vi "GetHGFunctionLookupTable.vi"(11 "G":dbl) -> (2 "Integrated Distribution":cluster{dbl[], dbl[]}(graph), 3 "Normalized Distribution":cluster{dbl[], dbl[]}(graph))   [LabVIEW 2019]
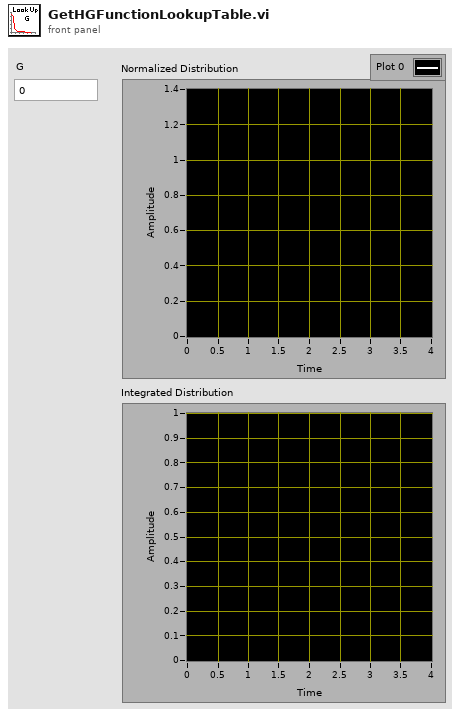
[diagram p1: front panel]
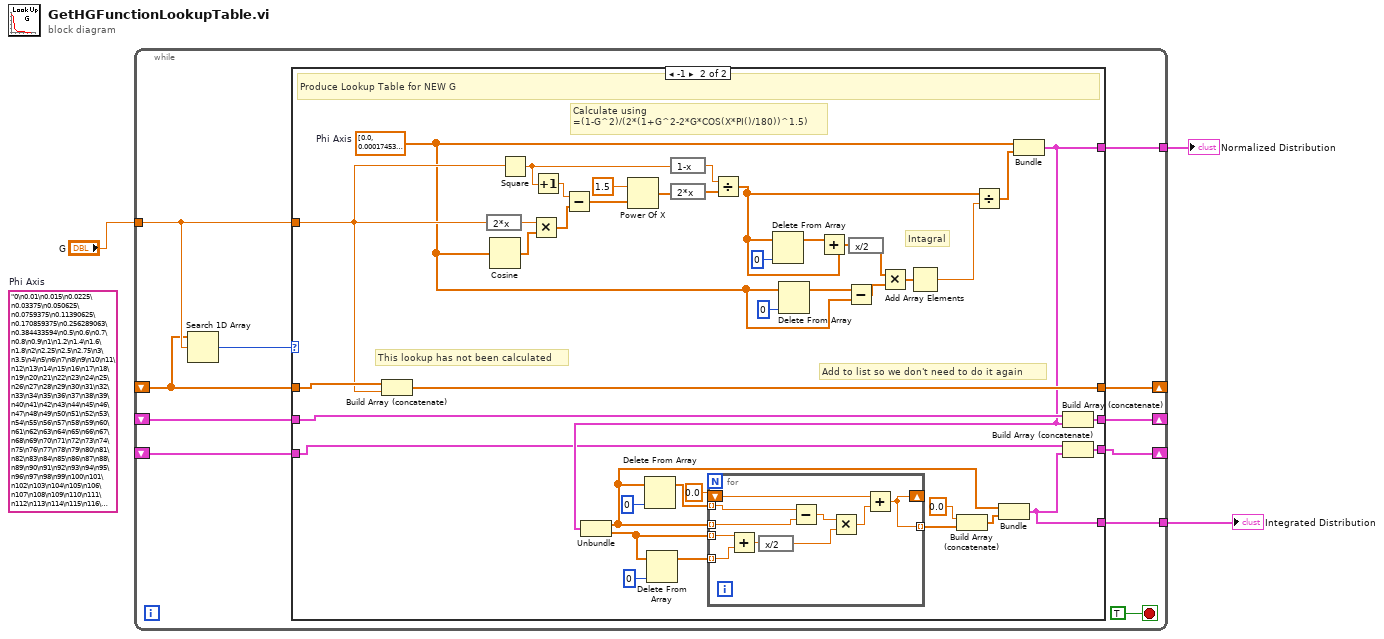
[diagram p0: block diagram]
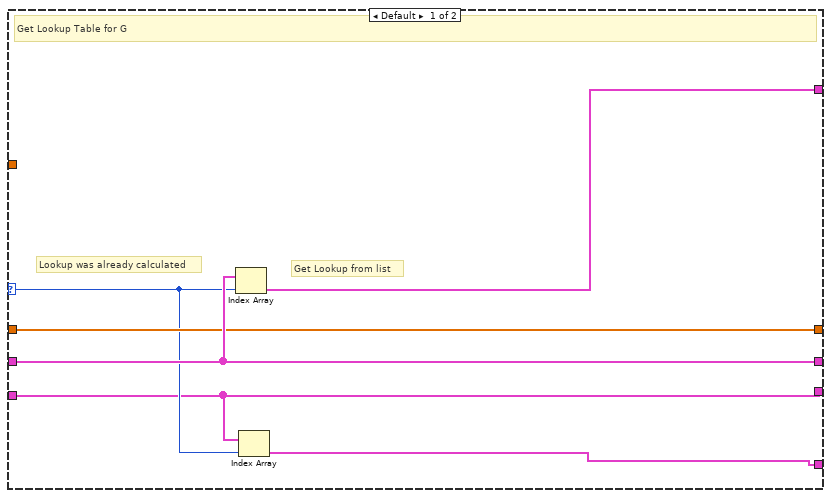
[diagram p2: hidden frame]
diagram:
  (unwired) "0\n0.01\n0.015\n0.0225\n0.03375\n0.050625\n0.0759375\n0.11390625\n0.170859375\n0.256289063\n0.384433594\n0.5\n0.6\n0.7\n0.8\n0.9\n1\n1.2\n1.4\n1.6\n1.8\n2\n2.25\n2.5\n2.75\n3\n3.5\n4\n5\n6\n7\n8\n9\n10\n11\n12\n13\n14\n15\n16\n17\n18\n19\n20\n21\n22\n23\n24\n25\n26\n27\n28\n29\n30\n31\n32\n33\n34\n35\n36\n37\n38\n39\n40\n41\n42\n43\n44\n45\n46\n47\n48\n49\n50\n51\n52\n53\n54\n55\n56\n57\n58\n59\n60\n61\n62\n63\n64\n65\n66\n67\n68\n69\n70\n71\n72\n73\n74\n75\n76\n77\n78\n79\n80\n81\n82\n83\n84\n85\n86\n87\n88\n89\n90\n91\n92\n93\n94\n95\n96\n97\n98\n99\n100\n101\n102\n103\n104\n105\n106\n107\n108\n109\n110\n111\n112\n113\n114\n115\n116\n117\n118\n119\n120\n121\n122\n123\n124\n125\n126\n127\n128\n129\n130\n131\n132\n133\n134\n135\n136\n137\n138\n139\n140\n141\n142\n143\n144\n145\n146\n147\n148\n149\n150\n151\n152\n153\n154\n155\n156\n157\n158\n159\n160\n161\n162\n163\n164\n165\n166\n167\n168\n169\n170\n171\n172\n173\n174\n175\n176\n177\n178\n179\n180\n"  # Phi Axis
  n1 = while {
    tunnel: [w14] -> w3
    shift-right: [w6] -> _
    shift-left: _ -> [w11]
    tunnel: "G" -> [w13]
    shift-right: [w5] -> _
    shift-left: _ -> [w10]
    tunnel: [w8] -> w1
    shift-right: [w4] -> _
    shift-left: _ -> [w7]
    stop <- TRUE stop-if-true
    n2 = Search 1D Array(1D array=w11, element=w13) -> (index of element=w12:i32)  [unwired: 1 in]
    n3 = case shown="-1" w12 {
      selector: w12 -> [w17 _]
      tunnel: [w20 w34] -> w14
      tunnel: w13 -> [_ w48]
      tunnel: w11 -> [w18 w50]
      tunnel: [w18 w49] -> w6
      tunnel: [w19 w47] -> w5
      tunnel: w10 -> [w19 w46]
      tunnel: [w15 w23] -> w8
      tunnel: [w16 w22] -> w4
      tunnel: w7 -> [w16 w21]
      frame Default {
        # "Get Lookup from list"
        # "Lookup was already calculated"
        # "Get Lookup Table for G"
        n4 = Index Array(array=w19, index=w17) -> (element=w20:cluster{"Phi Axis":dbl[], dbl[]})
        n5 = Index Array(array=w16, index=w17) -> (element=w15:cluster{"Phi Axis":dbl[], dbl[]})
      }
      frame -1 {
        w36 = dbl[] [0.0, 0.00017453292519943296, 0.0002617993877991494, 0.00039269908169872416, 0.0005890486225480862, 0.0008835729338221294, 0.001325359400733194, 0.001988039101099791, 0.0029820586516496866, 0.004473087986201175, 0.006709631970575117, 0.008726646259971648, 0.010471975511965976, 0.012217304763960306, 0.013962634015954637, 0.015707963267948967, 0.017453292519943295, 0.020943951023931952, 0.024434609527920613, 0.027925268031909273, 0.031415926535897934, 0.03490658503988659, 0.039269908169872414, 0.04363323129985824, 0.04799655442984406, 0.05235987755982988, 0.061086523819801536, 0.06981317007977318, 0.08726646259971647, 0.10471975511965977, 0.12217304763960307, 0.13962634015954636, 0.15707963267948966, 0.17453292519943295, 0.19198621771937624, 0.20943951023931953, 0.22689280275926285, 0.24434609527920614, 0.2617993877991494, 0.2792526803190927, 0.29670597283903605, 0.3141592653589793, 0.3316125578789226, 0.3490658503988659, 0.3665191429188092, 0.3839724354387525, 0.40142572795869574, 0.41887902047863906, 0.4363323129985824, 0.4537856055185257, 0.47123889803846897, 0.4886921905584123, 0.5061454830783556, 0.5235987755982988, 0.5410520681182421, 0.5585053606381855, 0.5759586531581288, 0.5934119456780721, 0.6108652381980153, 0.6283185307179586, 0.6457718232379019, 0.6632251157578452, 0.6806784082777885, 0.6981317007977318, 0.715584993317675, 0.7330382858376184, 0.7504915783575616, 0.767944870877505, 0.7853981633974483, 0.8028514559173915, 0.8203047484373349, 0.8377580409572781, 0.8552113334772214, 0.8726646259971648, 0.890117918517108, 0.9075712110370514, 0.9250245035569946, 0.9424777960769379, 0.9599310885968813, 0.9773843811168246, 0.9948376736367678, 1.0122909661567112, 1.0297442586766543, 1.0471975511965976, 1.064650843716541, 1.0821041362364843, 1.0995574287564276, 1.117010721276371, 1.1344640137963142, 1.1519173063162575, 1.1693705988362006, 1.1868238913561442, 1.2042771838760873, 1.2217304763960306, 1.239183768915974, 1.2566370614359172, 1.2740903539558606, 1.2915436464758039, 1.3089969389957472, 1.3264502315156903, 1.3439035240356338, 1.361356816555577, 1.3788101090755203, 1.3962634015954636, 1.413716694115407, 1.43116998663535, 1.4486232791552935, 1.4660765716752369, 1.4835298641951802, 1.5009831567151233, 1.5184364492350666, 1.53588974175501, 1.5533430342749535, 1.5707963267948966, 1.5882496193148399, 1.605702911834783, 1.6231562043547263, 1.6406094968746698, 1.6580627893946132, 1.6755160819145563, 1.6929693744344996, 1.710422666954443, 1.7278759594743864, 1.7453292519943295, 1.7627825445142729, 1.780235837034216, 1.7976891295541593, 1.8151424220741028, 1.8325957145940461, 1.8500490071139892, 1.8675022996339325, 1.8849555921538759, 1.902408884673819, 1.9198621771937625, 1.9373154697137058, 1.9547687622336491, 1.9722220547535922, 1.9896753472735356, 2.007128639793479, 2.0245819323134224, 2.0420352248333655, 2.0594885173533086, 2.076941809873252, 2.0943951023931953, 2.111848394913139, 2.129301687433082, 2.1467549799530254, 2.1642082724729685, 2.1816615649929116, 2.199114857512855, 2.2165681500327987, 2.234021442552742, 2.251474735072685, 2.2689280275926285, 2.286381320112572, 2.303834612632515, 2.321287905152458, 2.3387411976724013, 2.356194490192345, 2.3736477827122884, 2.3911010752322315, 2.4085543677521746, 2.426007660272118, 2.443460952792061, 2.4609142453120043, 2.478367537831948, 2.4958208303518914, 2.5132741228718345, 2.5307274153917776, 2.548180707911721, 2.5656340004316647, 2.5830872929516078, 2.600540585471551, 2.6179938779914944, 2.6354471705114375, 2.6529004630313806, 2.670353755551324, 2.6878070480712677, 2.705260340591211, 2.722713633111154, 2.740166925631097, 2.7576202181510405, 2.775073510670984, 2.792526803190927, 2.8099800957108703, 2.827433388230814, 2.844886680750757, 2.8623399732707, 2.8797932657906435, 2.897246558310587, 2.9146998508305306, 2.9321531433504737, 2.949606435870417, 2.9670597283903604, 2.9845130209103035, 3.0019663134302466, 3.01941960595019, 3.036872898470133, 3.0543261909900763, 3.07177948351002, 3.0892327760299634, 3.106686068549907, 3.12413936106985, 3.141592653589793]  # Phi Axis
        # "Intagral"
        # "Add to list so we don't need to do it again"
        # "This lookup has not been calculated"
        # "Calculate using\n=(1-G^2)/(2*(1+G^2-2*G*COS(X*PI()/180))^1.5)"
        # "Produce Lookup Table for NEW G"
        n6 = Build Array (concatenate)(w50, w48) -> (w49:dbl[])
        n7 = expression code="2*x"(w48) -> (w59:dbl)
        n8 = Cosine(x=w36) -> (cos(x)=w58:dbl[])
        n9 = Square(x=w48) -> (x^2=w61:dbl)
        n10 = Multiply(x=w59, y=w58) -> (x*y=w57:dbl[])
        n11 = Increment(x=w61) -> (x+1=w60:dbl)
        n12 = Subtract(x=w60, y=w57) -> (x-y=w56:dbl[])
        n13 = Power Of X(1:w56, 2:1.5 ("x^2")) -> (0:w54:dbl[])
        n14 = expression code="1-x"(w61) -> (w53:dbl)
        n15 = expression code="2*x"(w54) -> (w52:dbl[])
        n16 = Divide(x=w53, y=w52) -> (x/y=w51:dbl[])
        n17 = Delete From Array(array=w51, index=0) -> (array with subset deleted=w43:dbl[])  [unwired: 1 in, 1 out]
        n18 = Delete From Array(array=w36, index=0) -> (array with subset deleted=w44:dbl[])  [unwired: 1 in, 1 out]
        n19 = Add(x=w43, y=w51) -> (x+y=w40:dbl[])
        n20 = Subtract(x=w44, y=w36) -> (x-y=w41:dbl[])
        n21 = expression code="x/2"(w40) -> (w39:dbl[])
        n22 = Multiply(x=w39, y=w41) -> (x*y=w38:dbl[])
        n23 = Add Array Elements(numeric array=w38) -> (sum=w37:dbl)
        n24 = Divide(x=w51, y=w37) -> (x/y=w35:dbl[])
        n25 = Bundle("Phi Axis"=w36, w35) -> (w34:cluster{"Phi Axis":dbl[], dbl[]})  [unwired: 1 in]
        n26 = Unbundle(w34) -> ("Phi Axis"=w27:dbl[], w32:dbl[])
        n27 = Delete From Array(array=w27, index=0) -> (array with subset deleted=w30:dbl[])  [unwired: 1 in, 1 out]
        n28 = Delete From Array(array=w32, index=0) -> (array with subset deleted=w29:dbl[])  [unwired: 1 in, 1 out]
        n29 = for {
          tunnel: w27 -> [w63] mode=indexing
          tunnel: w32 -> [w69] mode=indexing
          tunnel: w30 -> [w62] mode=indexing
          tunnel: w29 -> [w70] mode=indexing
          shift-right: [w64] -> _
          shift-left: 0.0 -> [w65]
          tunnel: [w64] -> w28 mode=indexing
          n30 = Add(x=w69, y=w70) -> (x+y=w71:dbl)
          n31 = expression code="x/2"(w71) -> (w67:dbl)
          n32 = Subtract(x=w62, y=w63) -> (x-y=w68:dbl)
          n33 = Multiply(x=w68, y=w67) -> (x*y=w66:dbl)
          n34 = Add(x=w65, y=w66) -> (x+y=w64:dbl)
        }
        n35 = Build Array (concatenate)(0.0, w28) -> (w25:dbl[])
        n36 = Bundle("Phi Axis"=w27, w25) -> (w23:cluster{"Phi Axis":dbl[], dbl[]})  [unwired: 1 in]
        n37 = Build Array (concatenate)(w46, w34) -> (w47:cluster{"Phi Axis":dbl[], dbl[]}[])
        n38 = Build Array (concatenate)(w21, w23) -> (w22:cluster{"Phi Axis":dbl[], dbl[]}[])
      }
    }
  }
  "Normalized Distribution" <- w3
  "Integrated Distribution" <- w1
